vi "Lockin Proccess.vi"(4 "First call":bool, 6 "CH index":i32, 7 "Harmonics":i32[](array[numeric]), 8 "Error In":errorcluster, 9 "Harmonic":i32=1, 10 "User configuration":T1={"Time constant"=0.0, "Signal channels"=[], "Group"="p", "X channel"="", "Live update"=TRUE, "Phases"=[], "Harmonics"=[]} {"Phases" scale=-180.0..180.0; "Time constant" min=1e-06 max=1.0 scale=1e-06..0.01 scale format="%#_6p"}, 11 "Signal file":path) -> (0 "Error Out":errorcluster, 1 "dt":dbl, 2 "XY Graph":cluster{dbl[], "Y":dbl[]}[](graph), 3 "Signal file out":path, 5 "Signal names":cluster{"Signal Name":string, string[]})   [LabVIEW 2024]
uses:
  LabActor/Post-Processors/Lockin Processor/Lockin Processor Configuration.ctl
  Software Lock-in/Software Lock-in.lvclass
  <vilib>/express/express shared/transition.llb/Dynamic To Waveform Array.vi
  <vilib>/express/express signal manip/GetorSetDDTAttributes/Get DDT Attributes/Get DDT Properties.xnode
panel:
  out "Resample ref":dynamicdata(graph)
  out "Non-resampled signal":dynamicdata(graph)
  out "Attempts out":i32
  out "group":string
  out "owner":string
  out "permissions":i16
  out "Deleted channels":string[](array[string])
  out "Resampled signal":dynamicdata(graph)
  out "Resampled Y":dynamicdata(graph)
  out "Resampled X":dynamicdata(graph)
  in  "Save output":bool=TRUE
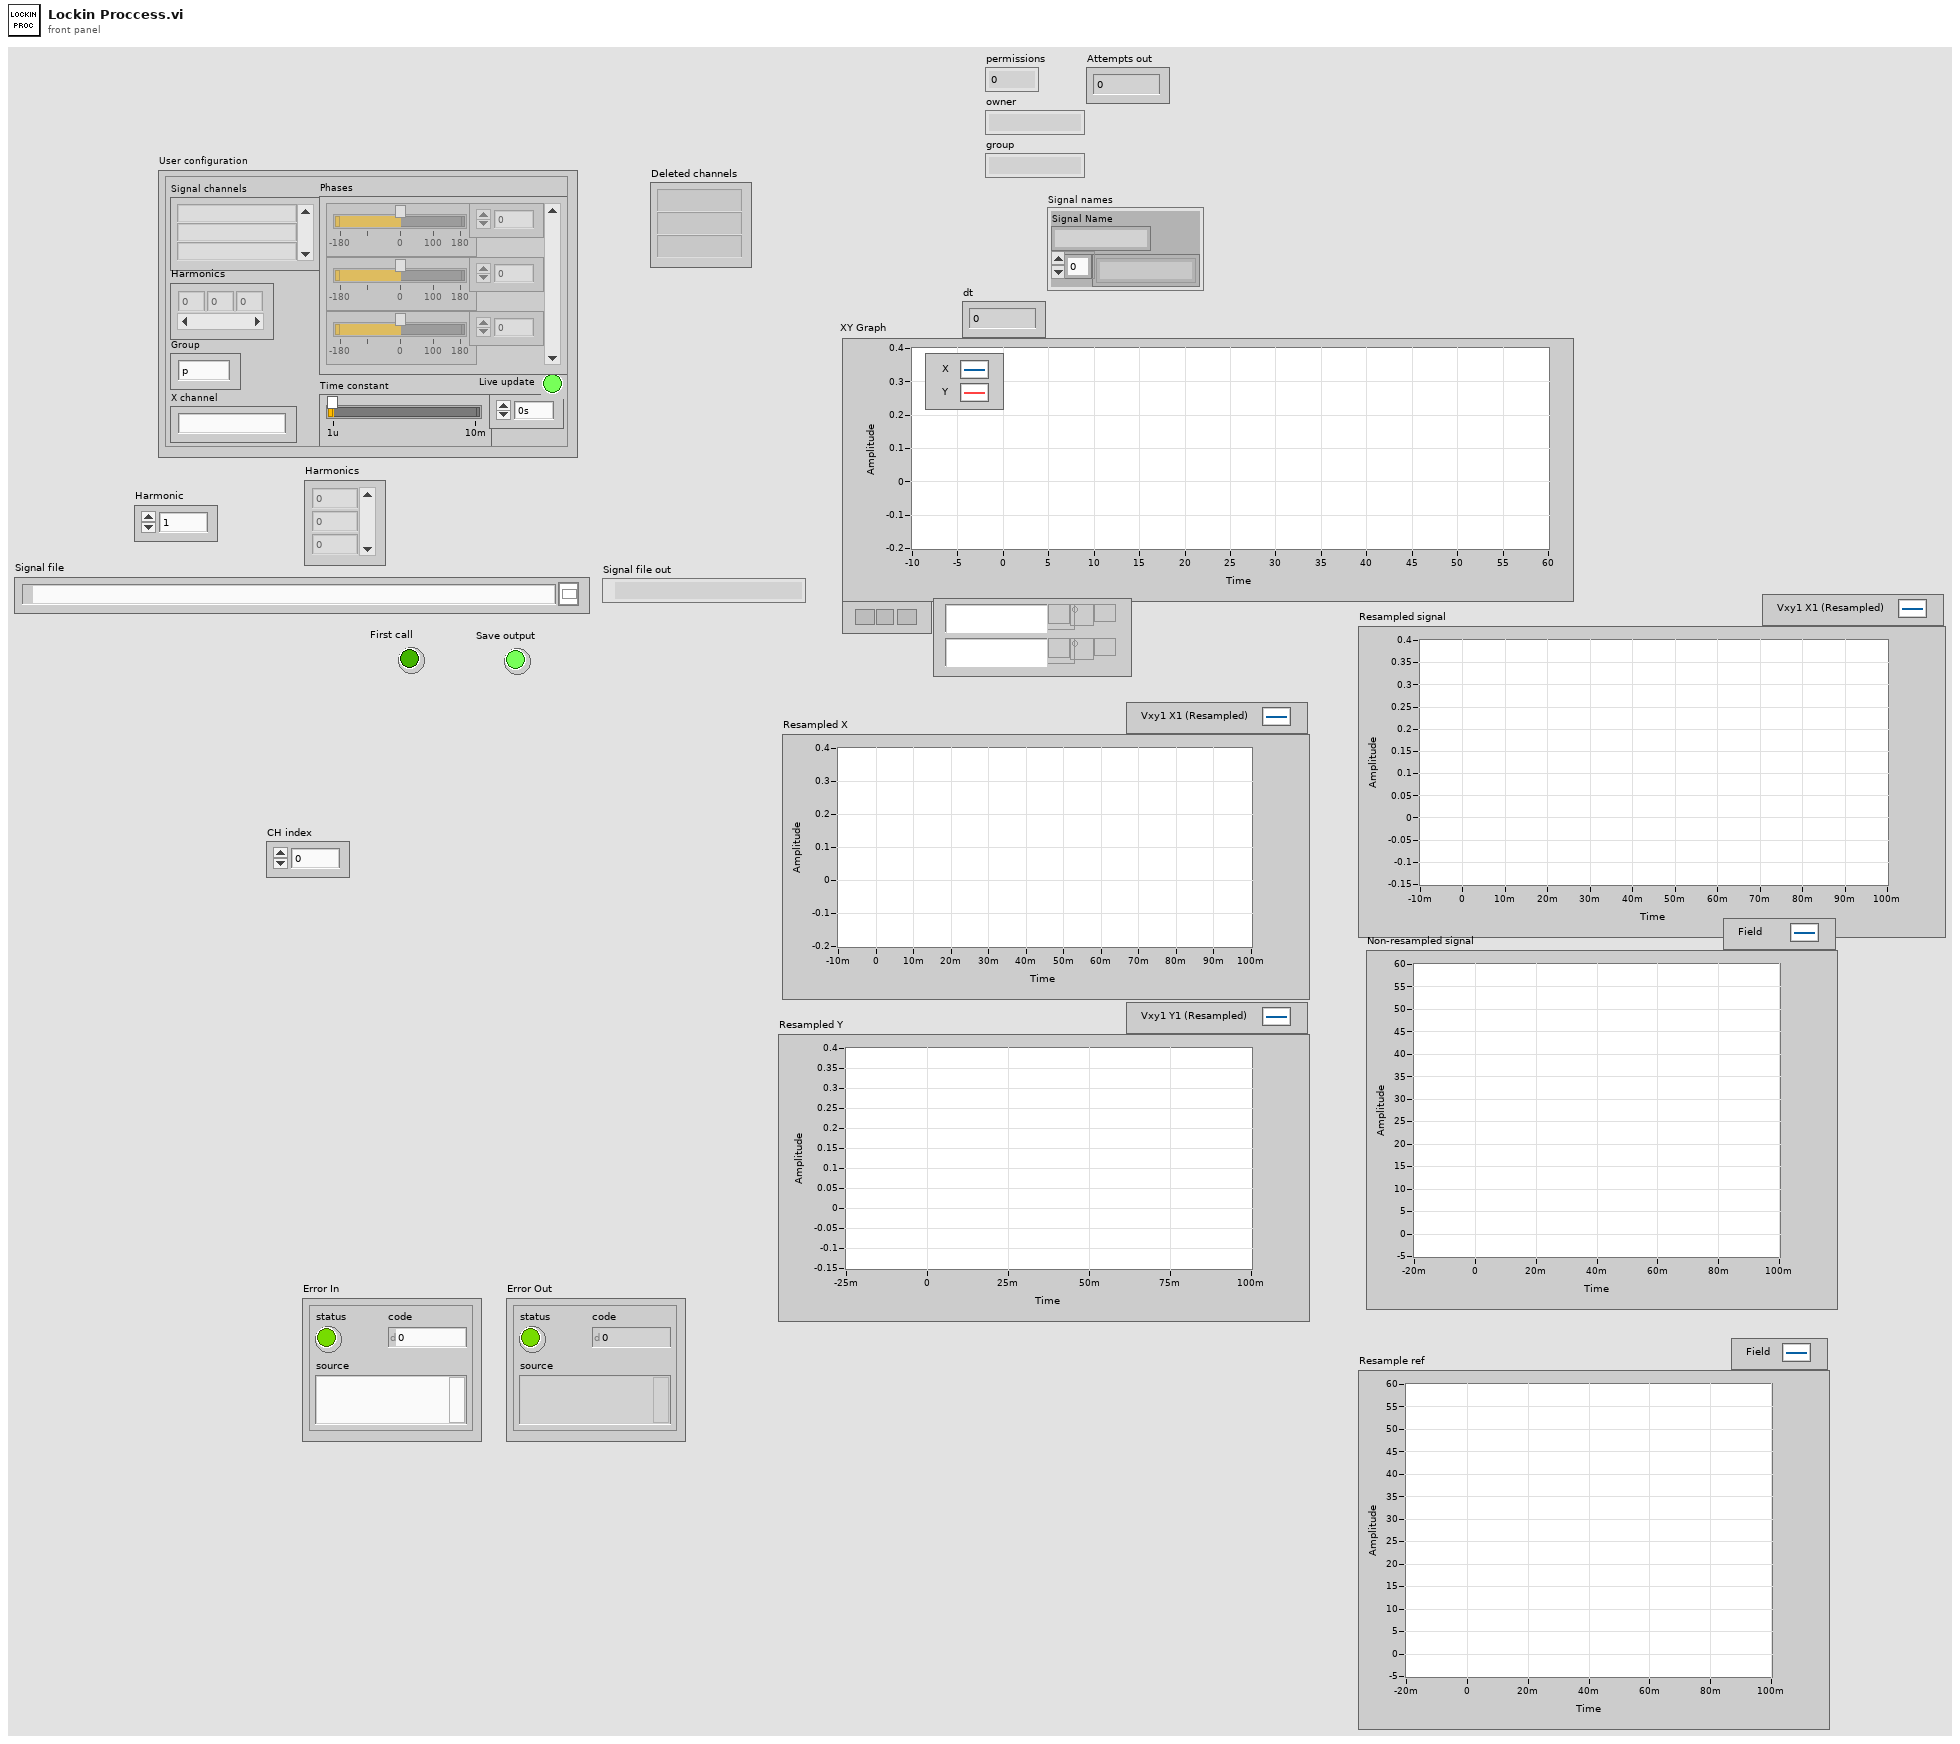
[diagram p1: front panel]
types:
  T1 = typedef "Lockin Processor Configuration.ctl" = cluster{"Time constant":dbl, "Signal channels":string[], "Group":string, "X channel":string, "Live update":bool, "Phases":dbl[], "Harmonics":i32[]}
  T2 = enum16{"open", "open or create", "create or replace", "create", "open (read-only)"}
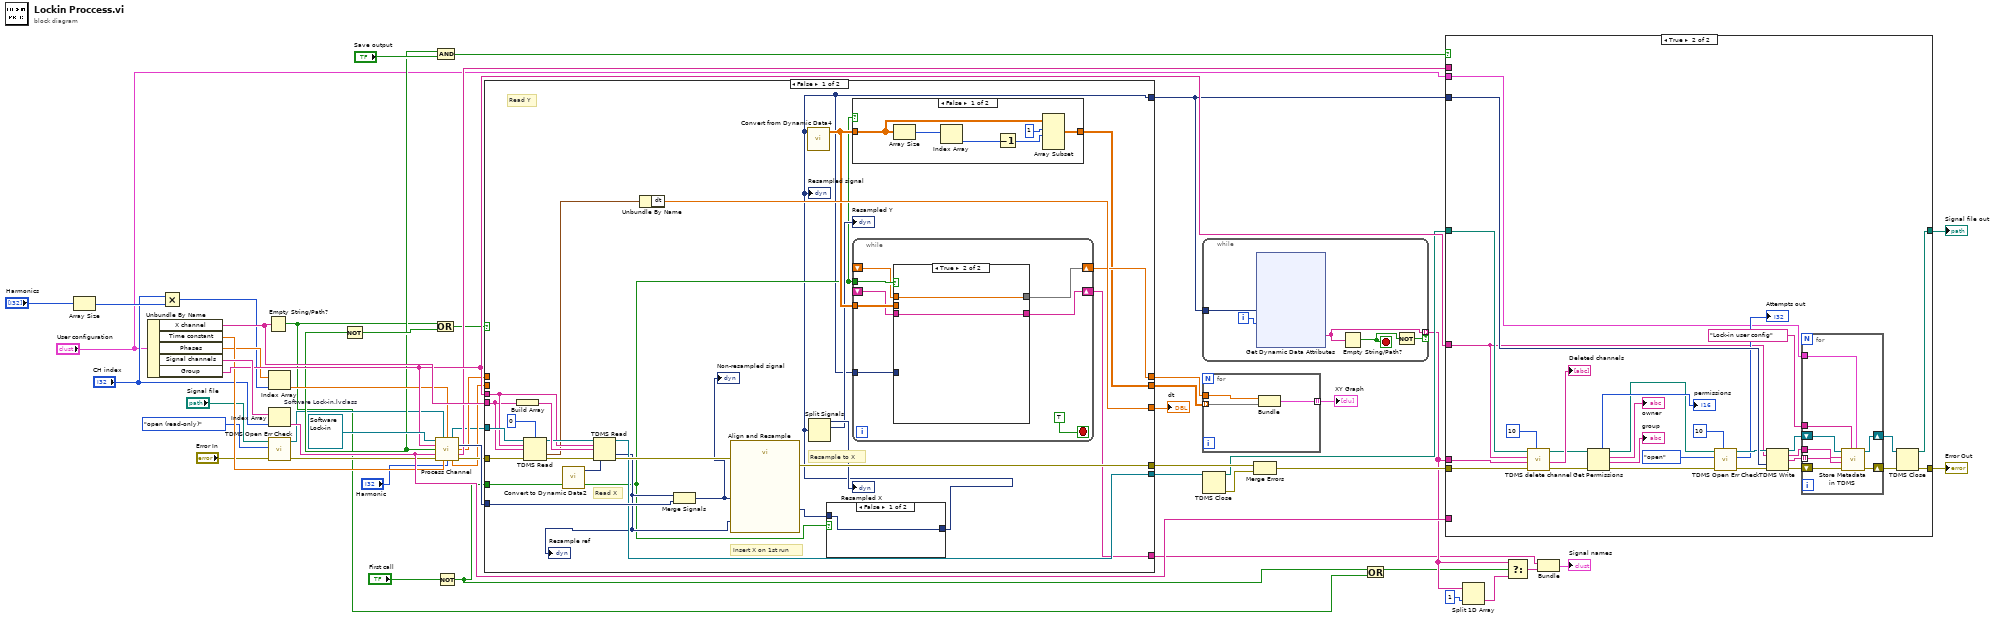
[diagram p0: block diagram]
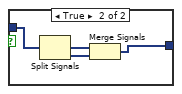
[diagram p2: hidden frame]
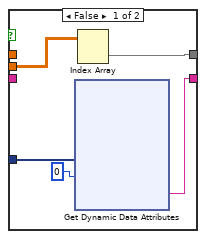
[diagram p4: hidden frame]
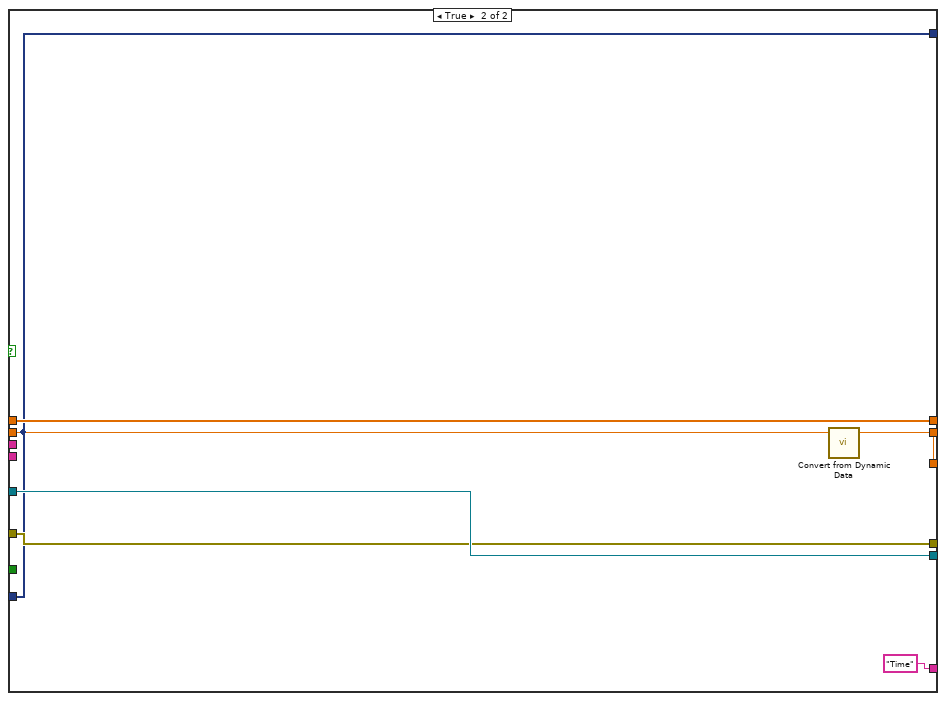
[diagram p5: hidden frame]
diagram:
  w46 = refnum<class "Software Lock-in.lvclass"> refnum  # Software Lock-in.lvclass
  n1 = Array Size(array="Harmonics") -> (size(s)=w16:i32)
  n2 = Unbundle By Name("User configuration") -> ("X channel"=w49:string, "Time constant"=w43:dbl, "Phases"=w23:dbl[], "Signal channels"=w50:string[], "Group"=w45:string)
  n3 = Multiply(x="CH index", y=w16) -> (x*y=w15:i32)
  n4 = Empty String/Path?(string/path=w49) -> (empty?=w2:bool)
  n5 = Index Array(array=w23, index=w15) -> (element=w20:dbl)
  n6 = Index Array(array=w50, index="CH index") -> (element=w44:string)
  n7 = call "TDMS Open Err Check.vi"("Error In"="Error In", "operation (0:open)"=T2."open (read-only)", "File Path Control"="Signal file") -> ("Error Out"=w7:errorcluster, "tdms file out"=w5:refnum<k34>)  [unwired: 6 in, 1 out]
  n8 = call-dynamic "Process Channel.vi"("Software Lock-in in"=w46, "tdms file"=w5, "Phase"=w20, "Group name"=w45, "Channel name"=w44, "error in (no error)"=w7, "Time constant"=w43, "Harmonic"="Harmonic") -> ("tdms file out"=w22:refnum<k34>, "Signal"=w42:dynamicdata, "found"=w10:bool, "Time axis"=w30:dbl[], "Channel names"=w41:string[], "dt"=w33:dbl, "error out"=w38:errorcluster)  [unwired: 1 out]
  n9 = Not(x=w10) -> (.not. x?=w12:bool)
  n10 = Or(x=w2, y=w12) -> (x .or. y?=w13:bool)
  n11 = And(x=w10, y="Save output") -> (x .and. y?=w11:bool)
  n12 = Not(x="First call") -> (.not. x?=w1:bool)
  n13 = case shown="False" w13 {
    tunnel: w42 -> [w78 w117]
    tunnel: w38 -> [w67 w120]
    tunnel: [w76 w120] -> w47
    tunnel: w49 -> [w68 _]
    tunnel: w45 -> [w69 _]
    tunnel: [w53 w117] -> w29
    tunnel: w22 -> [w71 w121]
    tunnel: [w73 w121] -> w40
    tunnel: [w64 w119] -> w34
    tunnel: w33 -> [_ w119]
    tunnel: [w62 w118] -> w32
    tunnel: [w61 w116] -> w31
    tunnel: w30 -> [_ w118]
    tunnel: w1 -> [w55 _]
    tunnel: [w58 "Time"] -> w21
    frame False {
      # "Read Y"
      # "Read X"
      # "Resample to X"
      # "Insert X on 1st run"
      n14 = Build Array(w68) -> (w74:string[])
      n15 = TDMS Read(0:w71, 2:i64 0 ("count (-1: all)"), 5:w69, 7:w68, 11:w67) -> (4:w70:refnum<k34>, 10:w65:waveform(dbl), 15:w66:errorcluster)  [unwired: 3 in, 3 out]
      n16 = call "Convert to Dynamic Data2"() -> ("Dynamic Data Type"=w75:dynamicdata)  [unwired: 4 in]
      n17 = TDMS Read(0:w70, 5:w69, 7:w74, 11:w66, 12:w75) -> (4:w73:refnum<k34>, 10:w56:dynamicdata, 15:w77:errorcluster)  [unwired: 3 in, 3 out]
      "Resample ref" <- w56
      n18 = Unbundle By Name(w65) -> ("dt"=w64:dbl)
      n19 = Merge Signals(w56, w78) -> (w57:dynamicdata)
      "Non-resampled signal" <- w57
      n20 = call "Align and Resample"("Reference Signal"=w56, "error in (no error)"=w77, "Signals"=w57) -> ("error out"=w76:errorcluster, "Resampled Signals"=w54:dynamicdata)  [unwired: 6 in, 1 out]
      n21 = case shown="False" w55 {
        tunnel: w54 -> [w79 w83]
        tunnel: [w79 w80] -> w53
        frame False {
        }
        frame True {
          n22 = Split Signals(w83) -> (w82:dynamicdata, w81:dynamicdata)  [unwired: 3 in, 1 out]
          n23 = Merge Signals(w82, w81) -> (w80:dynamicdata)
        }
      }
      "Resampled signal" <- w53
      n24 = call "Convert from Dynamic Data4"("Dynamic Data Type"=w53) -> ("Array"=w63:dbl[][])  [unwired: 3 in]
      n25 = Split Signals(w53) -> (→"Resampled X":dynamicdata, →"Resampled Y":dynamicdata)  [unwired: 4 in, 2 out]
      n26 = case shown="False" w55 {
        tunnel: w63 -> [w89 w90]
        tunnel: [w84 w90] -> w61
        frame False {
          n27 = Array Size(array=w89) -> (size(s)=w85:i32[])
          n28 = Index Array(array=w85) -> (element=w86:i32)  [unwired: 1 in]
          n29 = Decrement(x=w86) -> (x-1=w87:i32)
          n30 = Array Subset(array=w89, index (row)=1 ("index"), length (row)=w87) -> (w84:dbl[][])  [unwired: 2 in]
        }
        frame True {
        }
      }
      n31 = while {
        tunnel: w63 -> [w98]
        shift-right: [w97] -> w62
        shift-left: _ -> [w94]
        tunnel: w55 -> [w95]
        shift-right: [w92] -> w58
        shift-left: _ -> [w91]
        tunnel: w53 -> [w93]
        stop <- TRUE stop-if-true
        n32 = case shown="True" w95 {
          tunnel: w98 -> [w103 _]
          tunnel: [w102 w114] -> w97
          tunnel: w94 -> [_ w114]
          tunnel: w93 -> [w101 _]
          tunnel: [w99 w113] -> w92
          tunnel: w91 -> [_ w113]
          frame False {
            n33 = xnode "Get Dynamic Data Attributes"("Signals In"=w101, "Signal Index"=0) -> ("Signal Name"=w99:string)  [unwired: 1 in, 2 out]
            n34 = Index Array(array=w103) -> (element=w102:dbl[])  [unwired: 2 in]
          }
          frame True {
          }
        }
      }
    }
    frame True {
      n35 = call "Convert from Dynamic Data"("Dynamic Data Type"=w117) -> ("Array"=w116:dbl[][])  [unwired: 3 in]
    }
  }
  "dt" <- w34
  n36 = while {
    tunnel: w29 -> [w126]
    tunnel: [w124] -> w26 mode=indexing if=w122
    i -> [w125]
    stop <- w123 stop-if-true
    n37 = xnode "Get Dynamic Data Attributes"("Signals In"=w126, "Signal Index"=w125) -> ("Signal Name"=w124:string)  [unwired: 1 in, 2 out]
    n38 = Empty String/Path?(string/path=w124) -> (empty?=w123:bool)
    n39 = Not(x=w123) -> (.not. x?=w122:bool)
  }
  n40 = for {
    tunnel: w32 -> [w138]
    tunnel: w31 -> [w137] mode=indexing
    tunnel: [w136] -> w37 mode=indexing
    n41 = Bundle("Time axis"=w138, "Array"=w137) -> (w136:cluster{"Time axis":dbl[], "Array":dbl[]})  [unwired: 1 in]
  }
  "XY Graph" <- w37
  n42 = TDMS Close(11:w40) -> (0:w35:errorcluster, 3:w39:path)  [unwired: 1 in]
  n43 = Merge Errors(w47, w35) -> (w36:errorcluster)
  n44 = Or(x=w1, y=w2) -> (x .or. y?=w3:bool)
  n45 = case shown="True" w11 {
    tunnel: w39 -> [w139 w168]
    tunnel: w36 -> [w140 w167]
    tunnel: [w140 w169] -> w51
    tunnel: w44 -> [_ _]
    tunnel: w45 -> [_ w144]
    tunnel: [w139 w166] -> w48
    tunnel: w29 -> [_ w165]
    tunnel: w41 -> [_ _]
    tunnel: w26 -> [_ w164]
    tunnel: "User configuration" -> [_ w145]
    frame False {
    }
    frame True {
      n46 = call "TDMS delete channel.vi"("Delay"=u32 10, "error in (no error)"=w167, "Channels"=w164, "group name"=w144, "file path"=w168) -> ("error out"=w160:errorcluster, "Deleted channels"=→"Deleted channels":string[], "file path out"=w161:path)  [unwired: 4 in]
      n47 = Get Permissions(8:w160, 11:w161) -> (0:w156:errorcluster, 1:→"group":string, 2:→"owner":string, 3:w155:path, 5:→"permissions":i16)
      n48 = call "TDMS Open Err Check.vi"("Retry attempts"=10, "Error In"=w156, "operation (0:open)"=T2."open", "File Path Control"=w155) -> ("Error Out"=w152:errorcluster, "Attempts out"=→"Attempts out":i32, "tdms file out"=w153:refnum<k34>)  [unwired: 5 in]
      n49 = TDMS Write(0:w153, 5:w144, 9:w165, 11:w152) -> (4:w149:refnum<k34>, 6:w141:string, 8:w143:string[], 15:w147:errorcluster)  [unwired: 2 in]
      n50 = for {
        tunnel: w145 -> [w173]
        shift-right: [w176] -> w148
        shift-left: w149 -> [w177]
        shift-right: [w174] -> w146
        shift-left: w147 -> [w175]
        tunnel: w143 -> [w172] mode=indexing
        tunnel: "Lock-in user config" ("Name") -> [w170]
        tunnel: w141 -> [w171]
        n51 = call "Store Metadata in TDMS.vi"("Value"=w173, "name"=w170, "Error In"=w175, "channel name"=w172, "group name"=w171, "tdms file"=w177) -> ("Error Out"=w174:errorcluster, "tdms file out"=w176:refnum<k34>)  [unwired: 1 in, 3 out]
      }
      n52 = TDMS Close(8:w146, 11:w148) -> (0:w169:errorcluster, 3:w166:path)
    }
  }
  "Error Out" <- w51
  "Signal file out" <- w48
  n53 = Split 1D Array(array=w26, index=1) -> (second subarray=w27:string[])  [unwired: 1 out]
  n54 = Select(t=w26, s=w3, f=w27) -> (s? t:f=w25:string[])
  n55 = Bundle("Signal Name"=w21, w25) -> (→"Signal names":cluster{"Signal Name":string, string[]})  [unwired: 1 in]
